vi "Launch control engine.vi"(6 "colorMap":string, 8 "Error in":errorcluster, 9 "grouping":string, 10 "Rules String":string, 11 "Controlled VI":refnum<vi>) -> (0 "Error out":errorcluster, 2 "Exit event":refnum<user-event>, 3 "Refresh event":refnum<user-event>)   [LabVIEW 2019, in "LSS.lvlib"]
doc: "This VI launches the Property Control Engine for LSS. The Property Control Engine will monitor the state of certain controls based on the Rules String input and then control the style of the controls based on the values it finds. The property control engine is currently only compatible with Value Change events for controls. \n\n<b>Inputs:</b>\n<b>Controlled VI</b> - This reference should be to the VI that will be controlled by the LSS Engine. The user may launch as many LSS engines as desired, but must use one LSS engine per VI that will be controlled.\n<b>Rules String</b> - The Rules String defines the behaviors that the Property Control Engine is searching for, and the resulting effects that rule will cause. It is formatted as follows:\n\nIF NAME_OF_THE_CONTROL CONDITION VALUE\nTHEN LSS\nELSE LSS\n\nWhere NAME_OF_THE_CONTROL is a string that matches the label value of the conrol.\nCONDITION is one of the following ==, !=, <, >, >=, <=\nVALUE is the value that shall be used to compare against the value of the control. This\ncould be a string comparison of data or numberic comparison of value. It will also work\nfor enums so long as the comparison for the enum is against the numeric representation \nof the enum.\nTHEN is where the LSS goes that will be applied if the condition evaluates true. \nELSE is where the LSS goes that will be applied if the condition evaluates false. The else\nstatement is optional.\nLSS is the cascading Layout & Style Sheet that will be applied. See one of the LSS examples\nfor details on formatting of the LSS\n\n<b>colorMap</b> - This string is an LSS formatted string that allows the mapping of hexidecimal color constants to string names that are easier to remember. Once a color is defined in the colorMap, any subsequent LSS call can simply use the name of the color instead of the hexidecimal representation. The format for this string is as follows:\n colorMap{\n myColorName:#000000;\n}\n<b>grouping</b> - Style sheet determining how objects will be grouped. The format of the style sheet for grouping objects is as follows:\ngrouping{\n objectGroupName:frontPanelObjectName;\n objectGroupName2:frontPanelObjectName2;\n}\nWhere the specifier grouping must stay the same. objectGroupName is the name of the group, for example \"Group 1\". frontPanelObjectName is the name of the item on the front panel, for example \"Stop Button\". To add two buttons to group alpha would look as follows:\ngrouping{\n group alpha:Start Button;\n group alpha:Stop Button;\n}\n<b>Error In</b> - Error input terminal\n\n<b>Outputs:</b>\n<b>Refresh event</b> - Since the Property Control Engine is only capable of firing when a value change event occurs, this event can be used to force a set of properties to update without a value change event. This is equivelent to the \"Value Signaling\" event, without actually changing the value. The data expected by this event is the refnum of the control whose \"Rules\" should be checked again. For example, if you had a button that controlled 6 different properties, then something else changed somet of those properties and you wanted to re-evaluate the button again without actually clicking the button, use the refresh event. Alternatively if you pass an invalid reference (blank) to the event, it will refresh all rules.\n<b>Exit event</b> - The property control engine is asynchronously launched, and therefore running in the background. Use this event to terminate the property control engine when the calling VI is finished running. If this event is not fired, the property control engine will continue to run in the background.\n<b>Error Out</b> - Error output terminal"
uses:
  LSS.lvlib
  <vilib>/Utility/traverseref.llb/TRef TravTarget.ctl
  <vilib>/Utility/traverseref.llb/VI Scripting - Traverse.lvlib
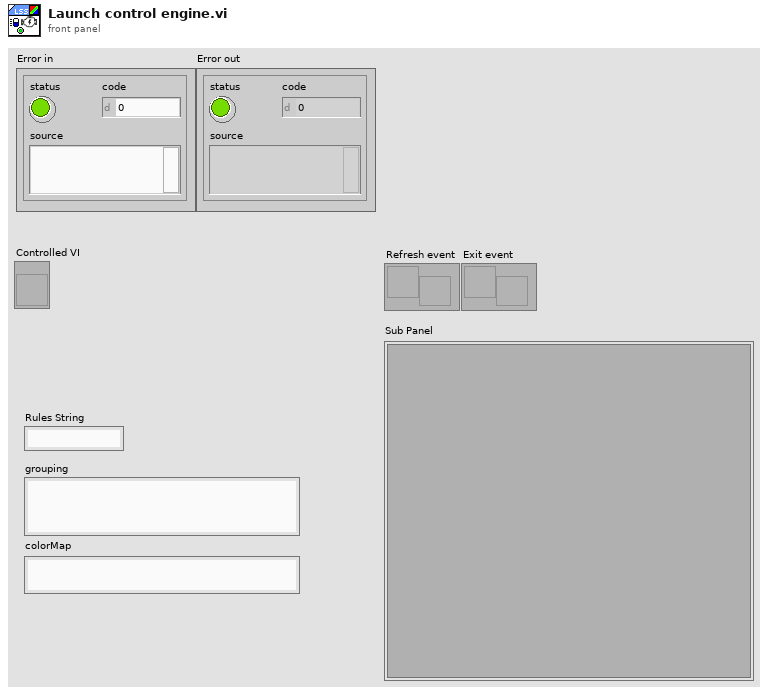
[diagram p1: front panel]
types:
  T1 = typedef "TRef TravTarget.ctl" = enum16{"FP", "BD", "Other"}
  T2 = enum32{"Invalid", "Standard", "Closed", "Hidden", "Minimized", "Maximized"}
  T3 = typedef "LSS.lvlib/Rule.ctl" = cluster{"Criteria":T4[], "Effects":T6[]}
  T4 = typedef "LSS.lvlib/Criteria.ctl" = cluster{"Name":string, "Comparison":T5, "Value":variant, "Operation":enum16{"Stack", "&&", "||"}}
  T5 = typedef "LSS.lvlib/Comparison Types.ctl" = enum16{"==", "!=", "<", ">", "<=", ">="}
  T6 = typedef "LSS.lvlib/Effects.ctl" = cluster{"Name":string, "CSS":string, "Apply when":bool}
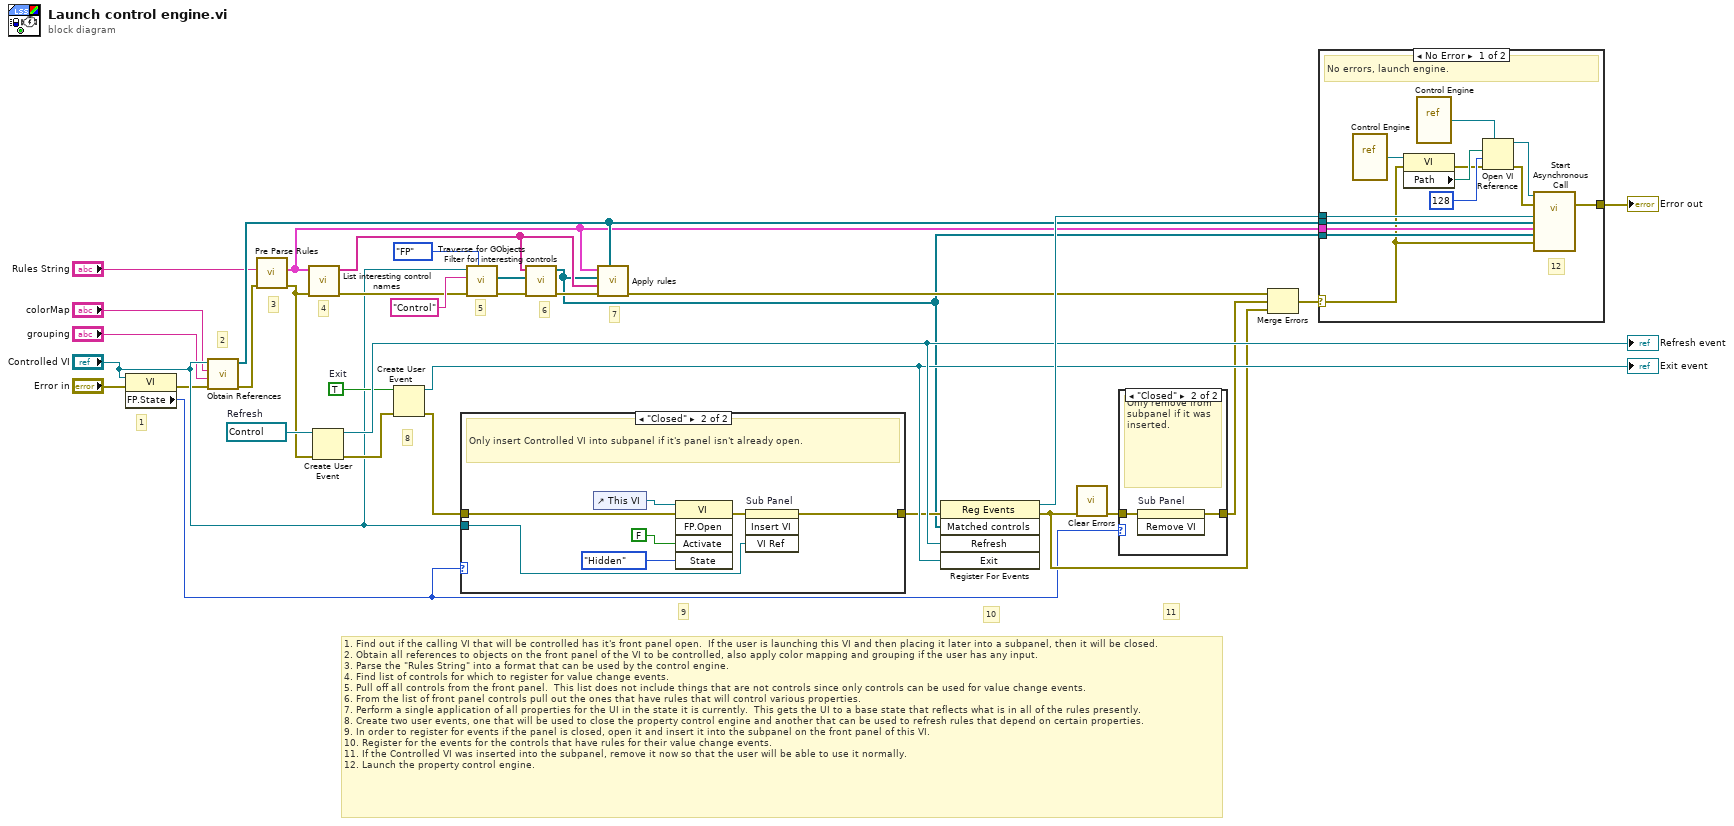
[diagram p0: block diagram]
diagram:
  w25 = TRUE  # Exit
  w26 = refnum<vi> refnum  # Refresh
  # "1. Find out if the calling VI that will be controlled has it's front panel open.  If the user is launching this VI and then placing it later into a subpanel, then it will be closed.\n2. Obtain all references to objects on the front panel of the VI to be controlled, also apply color mapping and grouping if the user has any input.\n3. Parse the \"Rules String\" into a format that can be used by the control engine.\n4. Find list of controls for which to register for value change events.\n5. Pull off all controls from the front panel.  This list does not include things that are not controls since only controls can be used for value change events.\n6. From the list of front panel controls pull out the ones that have rules that will control various properties.\n7. Perform a single application of all properties for the UI in the state it is currently.  This gets the UI to a base state that reflects what is in all of the rules presently.\n8. Create two user events, one that will be used to close the property control engine and another that can be used to refresh rules that depend on certain properties.\n9. In order to register for events if the panel is closed, open it and insert it into the subpanel on the front panel of this VI.  \n10. Register for the events for the controls that have rules for their value change events.\n11. If the Controlled VI was inserted into the subpanel, remove it now so that the user will be able to use it normally.\n12. Launch the property control engine."
  # "11"
  # "10"
  # "9"
  # "8"
  # "7"
  # "6"
  # "5"
  # "4"
  # "3"
  # "2"
  # "1"
  n1 = property class="VI"(reference="Controlled VI", error in="Error in") -> (error out=w4:errorcluster, "FP.State"=w17:T2)  [unwired: 1 out]
  n2 = call "Obtain References.vi"("Error In"=w4, "grouping"="grouping", "colorMap"="colorMap", "VI in"="Controlled VI") -> ("Error Out"=w8:errorcluster, "Front Panel Objects"=w15:refnum<vi>[])  [unwired: 6 in]
  n3 = call "Pre Parse Rules.vi"("Error in"=w8, "Rules String"="Rules String") -> ("Error out"=w10:errorcluster, "Processed Rules"=w11:T3[])  [unwired: 8 in]
  n4 = call "List interesting control names.vi"("Error in"=w10, "Rules"=w11) -> ("Error out"=w28:errorcluster, "Relevant Controls"=w14:string[])  [unwired: 8 in]
  n5 = Create User Event(user event datatype=w26, error in=w10) -> (user event=w27:refnum<user-event>, error out=w23:errorcluster)
  "Refresh event" <- w27
  n6 = Create User Event(user event datatype=w25, error in=w23) -> (user event=w24:refnum<user-event>, error out=w20:errorcluster)
  "Exit event" <- w24
  n7 = case shown="\"Closed\"" w17 {
    tunnel: [w34 w41] -> w21
    tunnel: w20 -> [w34 w37]
    tunnel: "Controlled VI" -> [_ w35]
    frame Default {
      # "VI's front panel is already open, do not insert into subpanel."
    }
    frame "Closed" {
      # "Only insert Controlled VI into subpanel if it's panel isn't already open."
      n8 = control-ref of="This VI"() -> (w40:refnum<vi>)
      n9 = invoke class="VI" method="FP.Open"(reference=w40, error in=w37, "Activate"=FALSE ("Activate?"), "State"=T2."Hidden") -> (error out=w36:errorcluster)  [unwired: 1 in, 4 out]
      n10 = invoke on="Sub Panel" class="SubPnl" method="Insert VI"(error in=w36, "VI Ref"=w35) -> (error out=w41:errorcluster)  [unwired: 2 in, 3 out]
    }
  }
  n11 = call <vilib>:"Traverse for GObjects.vi"("Traverse Target"=TRef_TravTarget."FP", "error in (no error)"=w28, "Class Name"="Control", "VI Refnum"="Controlled VI") -> ("error out"=w31:errorcluster, "References"=w13:refnum<vi>[])  [unwired: 4 in, 2 out]
  n12 = call "Filter for interesting controls.vi"("Error in"=w31, "All FP control references"=w13, "Interesting control names"=w14) -> ("Error out"=w29:errorcluster, "Matched controls"=w12:refnum<vi>[])  [unwired: 7 in]
  n13 = call "Apply rules.vi"("All References"=w15, "Error in"=w29, "Relevant control names"=w14, "Relevant controls"=w12, "Rules to apply"=w11) -> ("Error out"=w22:errorcluster)  [unwired: 4 in]
  n14 = register-events(error in=w21, w12, w27, w24) -> (reference out=w33:refnum<event-registration>, error out=w18:errorcluster)  [unwired: 1 in]
  n15 = call <vilib>:"Clear Errors.vi"("error in (no error)"=w18) -> ("error out"=w19:errorcluster)  [unwired: 5 in, 1 out]
  n16 = case shown="\"Closed\"" w17 {
    tunnel: [w42 w44] -> w3
    tunnel: w19 -> [w42 w43]
    frame Default {
      # "VI was not inserted into subpanel, no need to remove it."
    }
    frame "Closed" {
      # "Only remove from subpanel if it was inserted."
      n17 = invoke on="Sub Panel" class="SubPnl" method="Remove VI"(error in=w43) -> (error out=w44:errorcluster)  [unwired: 2 in, 2 out]
    }
  }
  n18 = Merge Errors(w22, w3, w18) -> (w2:errorcluster)
  n19 = case shown="No Error" w2 {
    selector: w2 -> [w46 w58]
    tunnel: w33 -> [w57 _]
    tunnel: w15 -> [w49 _]
    tunnel: w12 -> [w48 _]
    tunnel: w11 -> [w47 _]
    tunnel: [w45 w58] -> w1
    frame No Error {
      # "12"
      # "No errors, launch engine."
      n20 = vi-ref "Control Engine.vi"() -> (w56:refnum<vi>)
      n21 = property class="VI"(reference=w56, error in=w46) -> (error out=w50:errorcluster, "Path"=w55:path)  [unwired: 1 out]
      n22 = vi-ref "Control Engine.vi"() -> (w52:refnum<vi>)
      n23 = Open VI Reference(type specifier VI Refnum (for type only)=w52, vi path=w55, options=128, error in (no error)=w50) -> (vi reference=w53:refnum<vi>, error out=w54:errorcluster)  [unwired: 2 in]
      n24 = call-by-ref "Start Asynchronous Call"(reference=w53, error in=w54, "All References"=w49, 8:"error in (no error)"=w46, "Matched controls"=w48, "Rules"=w47, "Event Registration Refnum in"=w57) -> (error out=w45:errorcluster)  [unwired: 6 in, 2 out]
    }
    frame Error {
      # "Don't start engine if errors occur in setup."
    }
  }
  "Error out" <- w1
